vi "Write Max resend.vi"(8 "error in (no error)":errorcluster, 10 "Max resend":i32=3, 11 "BaseDriver in":refnum<class "BaseDriver.lvclass">) -> (0 "error out":errorcluster, 3 "BaseDriver out":refnum<class "BaseDriver.lvclass">)   [LabVIEW 2013, in "BaseDriver.lvclass"]
doc: "Maximum number of times to resend a message if a transmission failed. If sending fails this many times, a timeout event is generated"
uses:
  BaseDriver.lvclass
  BaseDriver.lvclass/BaseDriver.ctl
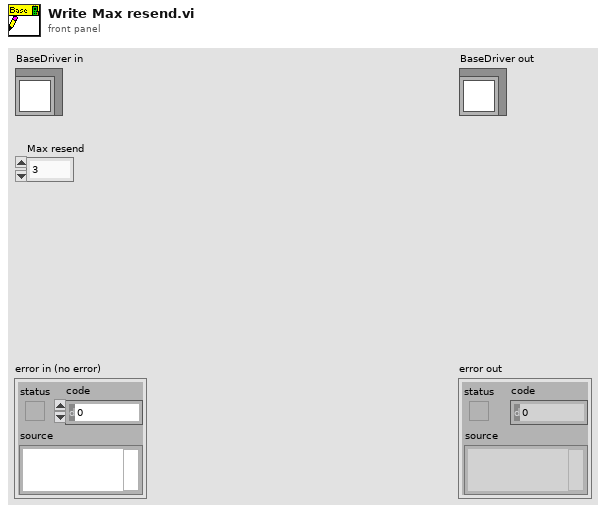
[diagram p1: front panel]
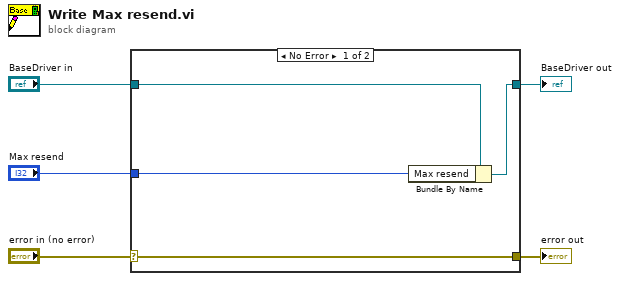
[diagram p0: block diagram]
diagram:
  n1 = case shown="No Error" "error in (no error)" {
    selector: "error in (no error)" -> [w9 w10]
    tunnel: [w9 w10] -> w4
    tunnel: [w7 w11] -> w2
    tunnel: "BaseDriver in" -> [w8 w11]
    tunnel: "Max resend" -> [w6 _]
    frame No Error {
      n2 = Bundle By Name(cluster=w8, "Max resend"=w6) -> (w7:refnum<class "BaseDriver.lvclass">)
    }
    frame Error {
    }
  }
  "error out" <- w4
  "BaseDriver out" <- w2
